vi "E7_28_readstring_2.vi"(7 "data string":string, 8 "error in":T9, 11 "DriverConnect in":T1={"InterfaceType"=enum."VISA", "OpenedSession"="", "InterfaceSettings"={"Interface"=enum."RS232", "EOS 4 read"=enum."LF (\\n)", "EOS 4 write"=enum."LF (\\n)", "TMO, ms"=10000, "Sett"=variant(cluster{"Baud Rate":u32, "Data Bits":u16, "Parity":u16, "Stop Bits":u16, "Flow Control":u16, "Eho":bool} {"Baud Rate"=75, "Data Bits"=0, "Parity"=0, "Stop Bits"=0, "Flow Control"=0, "Eho"=FALSE})}}) -> (0 "error out":T9, 3 "DriverConnect out":T1={"InterfaceType"=enum."VISA", "OpenedSession"="", "InterfaceSettings"={"Interface"=enum."RS232", "EOS 4 read"=enum."LF (\\n)", "EOS 4 write"=enum."LF (\\n)", "TMO, ms"=10000, "Sett"=variant(cluster{"Baud Rate":u32, "Data Bits":u16, "Parity":u16, "Stop Bits":u16, "Flow Control":u16, "Eho":bool} {"Baud Rate"=75, "Data Bits"=0, "Parity"=0, "Stop Bits"=0, "Flow Control"=0, "Eho"=FALSE})}}, 4 "Cluster 2":T6)   [LabVIEW 2018]
uses:
  MOKO_LabViewLibrary/MokoLowLevel/MokoLowLovelControl/MLLC_Error.ctl
  E7_28_DATA.ctl
  MOKO_LabViewLibrary/MokoLowLevel/MokoLowLovelControl/MLLC_Command.ctl
  MOKO_LabViewLibrary/MokoLowLevel/MokoLowLovelControl/MLLC_ErrorCode.ctl
  MOKO_LabViewLibrary/MokoLowLevel/MokoLowLovelControl/MLLC_ConnectCluster.ctl
  MOKO_LabViewLibrary/MokoLowLevel/MokoLowLovelControl/MLLC_InterfaceType.ctl
  MOKO_LabViewLibrary/MokoLowLevel/MokoLowLovelControl/MLLC_OpenedSession.ctl
  MOKO_LabViewLibrary/MokoLowLevel/MokoLowLovelControl/MLLC_InterfaceSettings.ctl
  MOKO_LabViewLibrary/MokoLowLevel/MokoLowLovelControl/MLLC_InterfaceKind.ctl
panel:
  out "Error answer string":string
  in  "input":u8=1 format="%b"
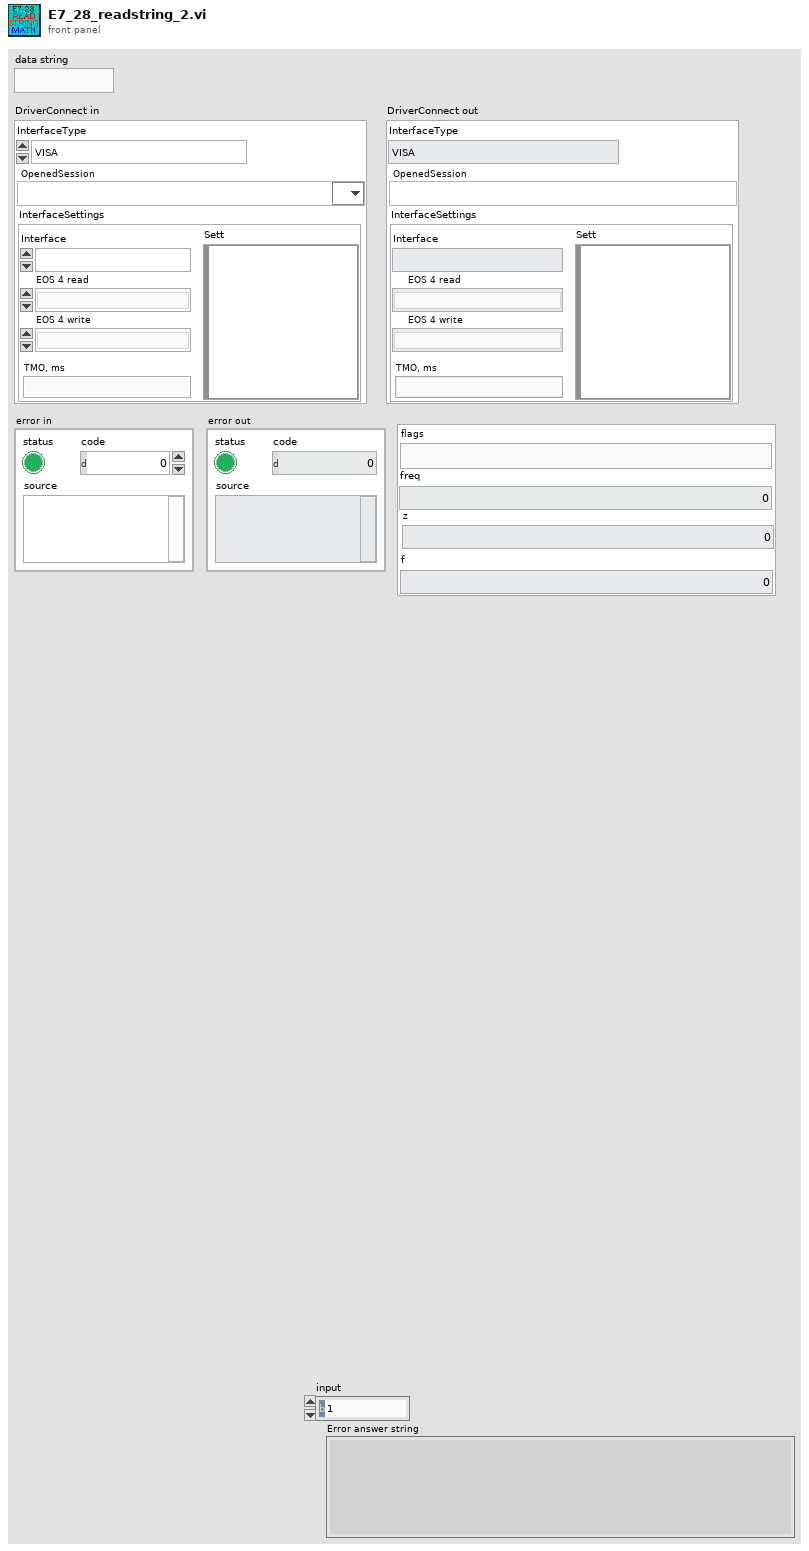
[diagram p1: front panel]
types:
  T1 = typedef "MLLC_ConnectCluster.ctl" = cluster{"InterfaceType":T2, "OpenedSession":T3, "InterfaceSettings":T4}
  T2 = typedef "MLLC_InterfaceType.ctl" = enum16{"VISA", "Prologix USB-GPIB"}
  T3 = typedef "MLLC_OpenedSession.ctl" = refnum<visa-resource-name>
  T4 = typedef "MLLC_InterfaceSettings.ctl" = cluster{"Interface":T5, "EOS 4 read":enum16{"Default (=EOS 4 write)", "CR (\\r)", "LF (\\n)", "None"}, "EOS 4 write":enum16{"CR+LF (\\r\\n)", "CR (\\r)", "LF (\\n)", "None"}, "TMO, ms":i32, "Sett":variant}
  T5 = typedef "MLLC_InterfaceKind.ctl" = enum16{"RS232", "GPIB", "USB", "Ethernet", "another"}
  T6 = typedef "E7_28_DATA.ctl" = cluster{"flags":T7, "freq":T8, "z":dbl, "f":T8}
  T7 = typedef "MLLC_Command.ctl" = string
  T8 = typedef "MLLC_ErrorCode.ctl" = u32
  T9 = typedef "MLLC_Error.ctl" = errorcluster
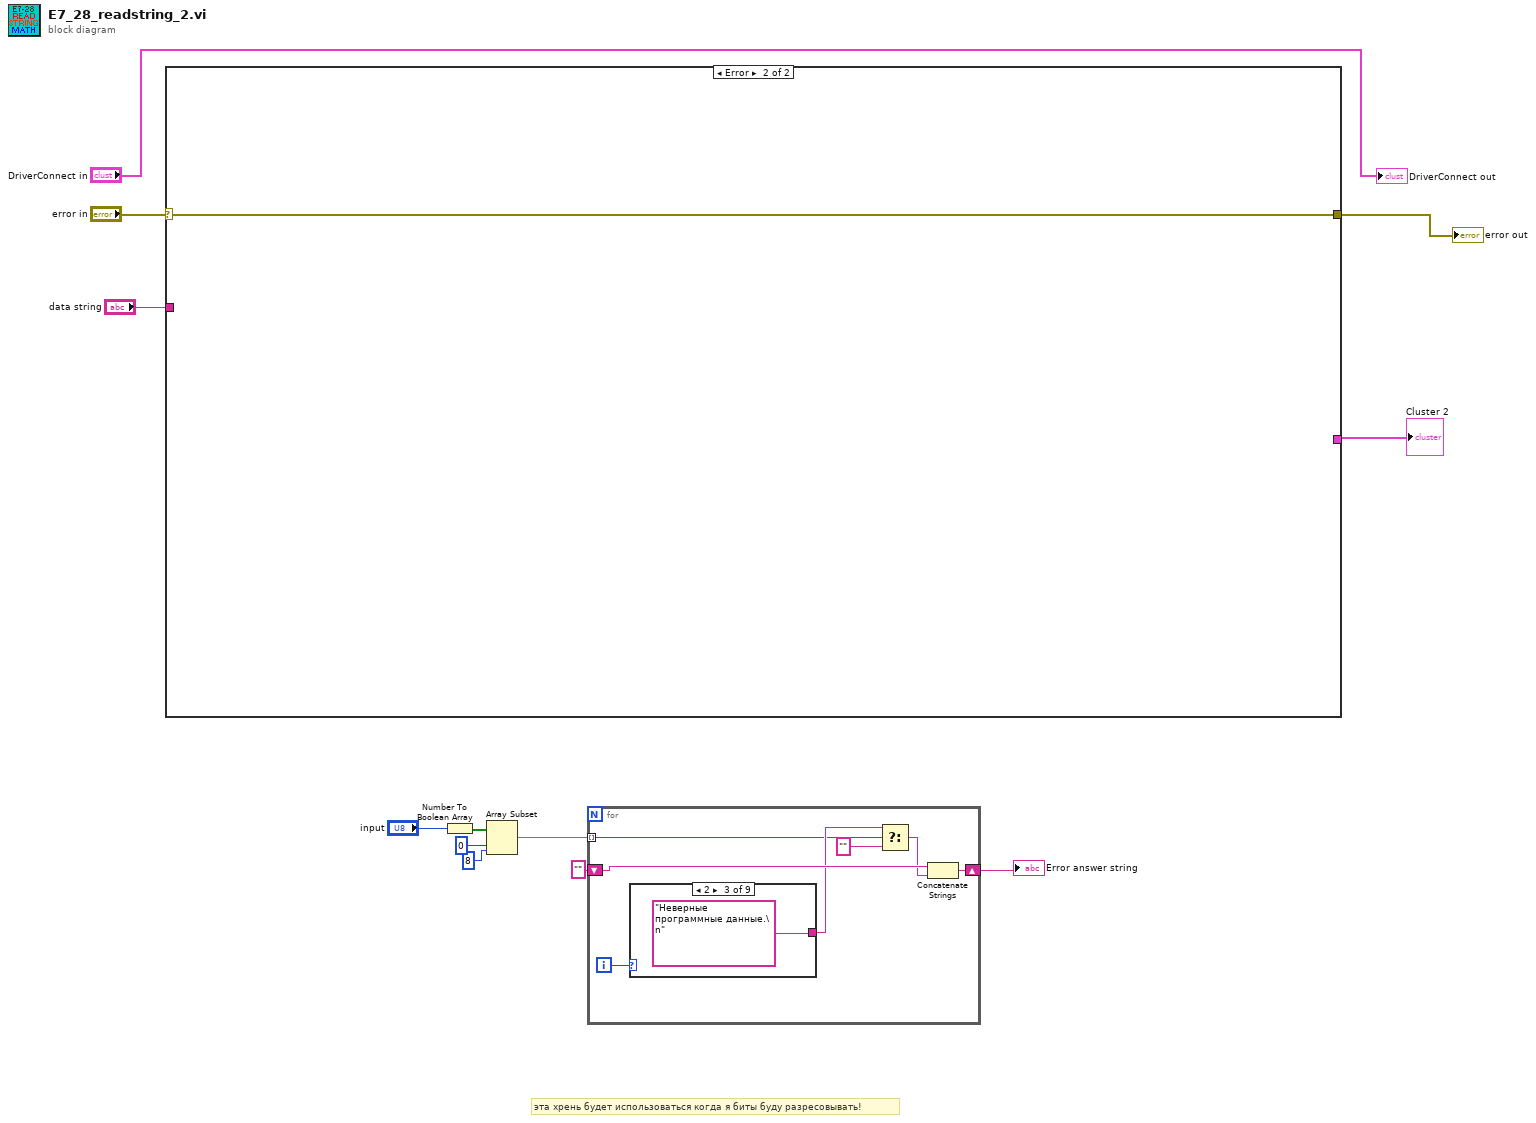
[diagram p0: block diagram]
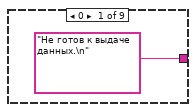
[diagram p2: hidden frame]
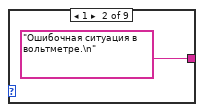
[diagram p3: hidden frame]
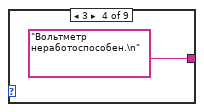
[diagram p4: hidden frame]
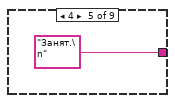
[diagram p5: hidden frame]
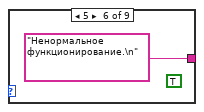
[diagram p6: hidden frame]
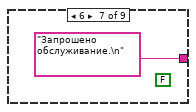
[diagram p7: hidden frame]
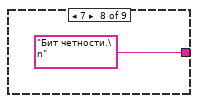
[diagram p8: hidden frame]
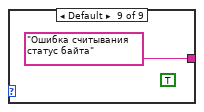
[diagram p9: hidden frame]
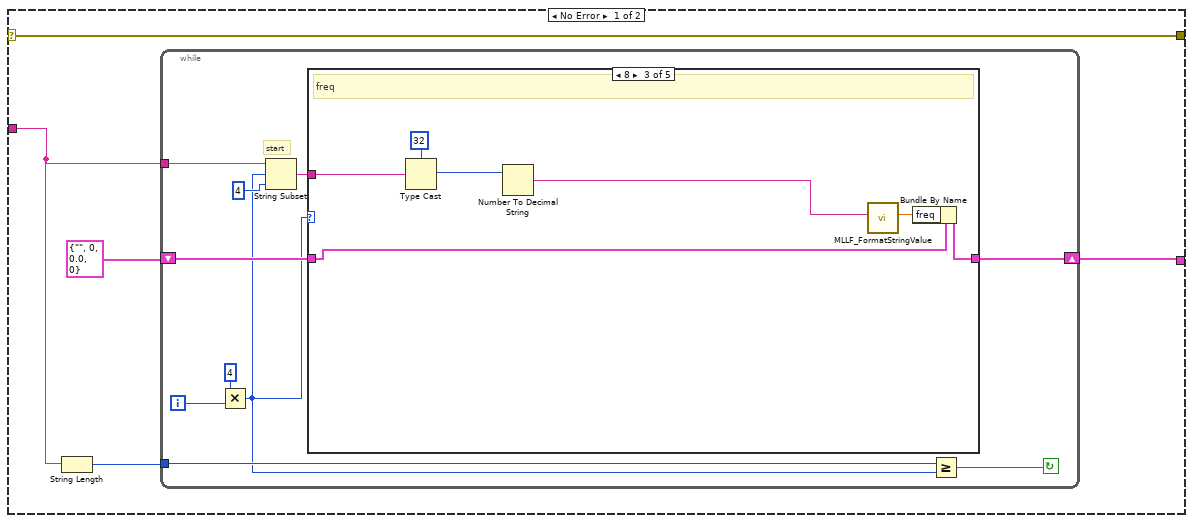
[diagram p10: hidden frame]
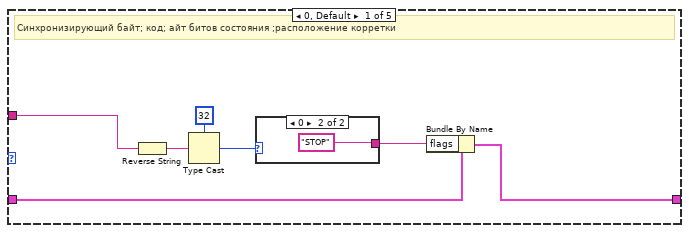
[diagram p11: hidden frame]
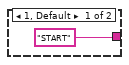
[diagram p12: hidden frame]
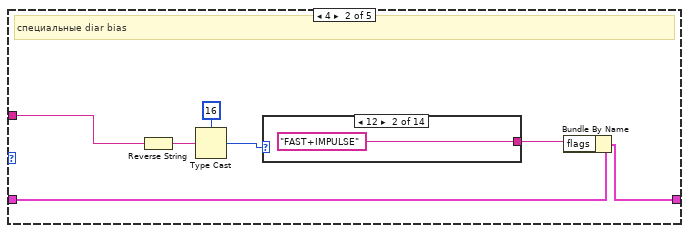
[diagram p13: hidden frame]
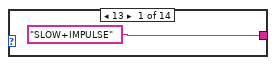
[diagram p14: hidden frame]
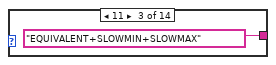
[diagram p15: hidden frame]
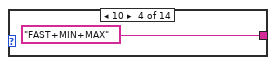
[diagram p16: hidden frame]
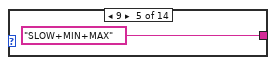
[diagram p17: hidden frame]
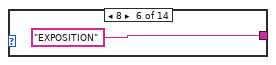
[diagram p18: hidden frame]
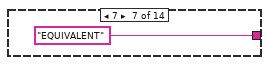
[diagram p19: hidden frame]
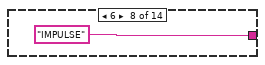
[diagram p20: hidden frame]
diagram:
  # "эта хрень будет использоваться когда я биты буду разресовывать!"
  n1 = case shown="Error" "error in" {
    selector: "error in" -> [w17 w77]
    tunnel: [w17 w77] -> w12
    tunnel: "data string" -> [w15 _]
    tunnel: [w13 _] -> w9
    frame No Error {
      n2 = String Length(string=w15) -> (length=w16:i32)
      n3 = while {
        tunnel: w15 -> [w25]
        tunnel: w16 -> [w24]
        shift-right: [w20] -> w13
        shift-left: T6 {"flags"="", "freq"=0, "z"=0.0, "f"=0} ("Cluster") -> [w19]
        i -> [w22]
        stop <- w23 continue-if-true
        # "start"
        n4 = Multiply(x=4, y=w22) -> (x*y=w18:i32)
        n5 = String Subset(string=w25, offset (0)=w18, length (rest)=4 ("length (rest)")) -> (substring=w21:string)
        n6 = case shown="8" w18 {
          tunnel: w21 -> [w31 w38 w60 w65 w73]
          tunnel: [w29 w42 w64 w68 w75] -> w20
          tunnel: w19 -> [w30 w43 w58 w69 w76]
          frame 0, Default {
            # "Синхронизирующий байт; код; айт битов состояния ;расположение корретки"
            n7 = Reverse String(1:w31) -> (0:w33:string)
            n8 = Type Cast(type=u32 32, x=w33) -> (*(type *) &x=w34:u32)
            n9 = case shown="0" w34 {
              tunnel: ["START" "STOP"] -> w28
              frame 1, Default {
              }
              frame 0 {
              }
            }
            n10 = Bundle By Name(cluster=w30, "flags"=w28) -> (w29:T6)
          }
          frame 4 {
            # "специальные diar bias"
            n11 = Reverse String(1:w38) -> (0:w40:string)
            n12 = Type Cast(type=u16 16, x=w40) -> (*(type *) &x=w39:u16)
            n13 = case shown="12" w39 {
              tunnel: ["SLOW+IMPULSE" "FAST+IMPULSE" "EQUIVALENT+SLOWMIN+SLOWMAX" "FAST+MIN+MAX" "SLOW+MIN+MAX" "EXPOSITION" "EQUIVALENT" "IMPULSE" "FASTMAX" "FASTMIN" "FAST" "SLOWMAX" "SLOWMIN" "SLOW"] -> w37
              frame 13 {
              }
              frame 12 {
              }
              frame 11 {
              }
              frame 10 {
              }
              frame 9 {
              }
              frame 8 {
              }
              frame 7 {
              }
              frame 6 {
              }
              frame 5 {
              }
              frame 4 {
              }
              frame 3 {
              }
              frame 2 {
              }
              frame 1 {
              }
              frame 0, Default {
              }
            }
            n14 = Bundle By Name(cluster=w43, "flags"=w37) -> (w42:T6)
          }
          frame 8 {
            # "freq"
            n15 = Type Cast(type=u32 32, x=w60) -> (*(type *) &x=w61:u32)
            n16 = Number To Decimal String(number=w61) -> (decimal integer string=w59:string)  [unwired: 1 in]
            n17 = call "MLLF_FormatStringValue.vi"("String Value"=w59) -> ("number"=w63:dbl)  [unwired: 8 in, 2 out]
            n18 = Bundle By Name(cluster=w58, "freq"=w63) -> (w64:T6)
          }
          frame 12 {
            # "SGL"
            # "float Z"
            n19 = Type Cast(type=sgl 0.0 ("32-bit IEEE 754"), x=w65) -> (*(type *) &x=w66:sgl)
            n20 = Bundle By Name(cluster=w69, "z"=w66) -> (w68:T6)
          }
          frame 16 {
            # "коэф перевода"
            # "SGL"
            # "float f"
            n21 = Type Cast(type=sgl 0.0 ("32-bit IEEE 754"), x=w73) -> (*(type *) &x=w72:sgl)
            n22 = Multiply(x=w72, y=57.2958) -> (x*y=w70:dbl)
            n23 = Bundle By Name(cluster=w76, "f"=w70) -> (w75:T6)
          }
        }
        n24 = Greater Or Equal?(x=w24, y=w18) -> (x >= y?=w23:bool)
      }
    }
    frame Error {
    }
  }
  "error out" <- w12
  "Cluster 2" <- w9
  n25 = Number To Boolean Array(number="input") -> (Boolean array=w8:bool[])
  n26 = Array Subset(array=w8, index=0, length=8) -> (w5:bool[])
  n27 = for {
    tunnel: w5 -> [w78] mode=indexing
    shift-right: [w82] -> w2
    shift-left: "" ("Driver Name") -> [w83]
    i -> [w84]
    n28 = case shown="2" w84 {
      tunnel: ["Не готов к выдаче данных.\n" ("Driver Name") "Ошибочная ситуация в вольтметре.\n" ("Driver Name") "Неверные программные данные.\n" ("Driver Name") "Вольтметр неработоспособен.\n" ("Driver Name") "Занят.\n" ("Driver Name") "Ненормальное функционирование.\n" ("Driver Name") "Запрошено обслуживание.\n" ("Driver Name") "Бит четности.\n" ("Driver Name") "Ошибка считывания статус байта" ("Driver Name")] -> w80
      frame 0 {
      }
      frame 1 {
      }
      frame 2 {
      }
      frame 3 {
      }
      frame 4 {
      }
      frame 5 {
        (unwired) TRUE
      }
      frame 6 {
        (unwired) FALSE
      }
      frame 7 {
      }
      frame Default {
        (unwired) TRUE
      }
    }
    n29 = Select(t=w80, s=w78, f="" ("Driver Name")) -> (s? t:f=w81:string)
    n30 = Concatenate Strings(w83, w81) -> (w82:string)
  }
  "Error answer string" <- w2
  "DriverConnect out" <- "DriverConnect in"
